vi "CANopen Emergency.vi"() -> ()   [LabVIEW 2016]
doc: "This example demonstrates how to read a CANopen emergency object."
uses:
  <vilib>/userdefined/High Color/nirio_resource_hc.ctl
  <vilib>/Platform/TimedLoop/XDataNode/timing_clust.ctl
  <vilib>/Platform/TimedLoop/XDataNode/nitl_modes.ctl
  <vilib>/Platform/TimedLoop/XDataNode/wakeup.ctl
  <vilib>/FPGAPlugInAG/cRIO-9033/niLvFpga_Open_cRIO-9033.vi
  <vilib>/rvi/interface/common/dynamic/niFpgaDynamicAddResources.vi
  <vilib>/CANopenLib/CANOPEN.llb/CANopen Interface Create.vi
  <vilib>/CANopenLib/CANOPEN.llb/CANopen Emergency Create.vi
  <vilib>/CANopenLib/CANOPEN.llb/CANopen Emergency Start.vi
  <vilib>/CANopenLib/CANOPEN.llb/CANopen Emergency Read.vi
  <vilib>/CANopenLib/CANOPEN.llb/CANopen Emergency Close.vi
  <vilib>/CANopenLib/CANOPEN.llb/CANopen Interface Close.vi
  <vilib>/FPGAPlugInAG/Dynamic/niLvFpga_Close_Dynamic.vi
  <vilib>/rvi/interface/nirviOpenFPGA/nirviOpenFPGA.xnode
  FPGA Bitfiles/project_FPGATarget_MainFPGA_S9ZLErdeBuw.lvbitx
  FPGA/MainFPGA.vi
  <vilib>/Platform/TimedLoop/XDataNode/XDataNode.xnode
  <vilib>/rvi/interface/nirviCloseFPGA/nirviCloseFPGA.xnode
  <vilib>/Platform/TimedLoop/XDataNode/XDNodeRunTimeDep.lvlib
panel:
  in  "error in":errorcluster
  out "emergency message":T1
  out "Is new?":bool
  out "timestamp":timestamp
  in  "stop":bool
  in  "period (ms)":i64=10
  in  "queue size":u16
  in  "node-ID":u8=1 min=1 max=127 step=1
  in  "baud rate":u32(ring)=2 items=["1 Mbit/s"=0, "800 kbit/s"=1, "500 kbit/s"=2, "250 kbit/s"=3, "125 kbit/s"=4, "50 kbit/s"=6, "20 kbit/s"=7, "10 kbit/s"=8]
  in  "CANopen interface":u32(ring) items=["CANopen01", "CANopen02", "CANopen03", "CANopen04", "CANopen05", "CANopen06", "CANopen07", "CANopen08", "CANopen09", "CANopen10", "CANopen11", "CANopen12", "CANopen13", "CANopen14", "CANopen15", "CANopen16", "CANopen17", "CANopen18", "CANopen19", "CANopen20", "CANopen21", "CANopen22", "CANopen23", "CANopen24", "CANopen25", "CANopen26", "CANopen27", "CANopen28", "CANopen29", "CANopen30", "CANopen31", "CANopen32"]
  # "Overview: This example demonstrates how to read a CANopen Emergency object.\nRequirements: Connect CANopen module with a slave device. \nInstructions: \n1. Specify the values of CANopen interface, baud rate of the CANopen interface, node-ID of the slave device and\n    queue size of Emergency object. \n2. Run this VI.\n3. Click STOP to stop the VI."
  # "Create CANopen interface and Emergency object"
  # "Read Emergency messages"
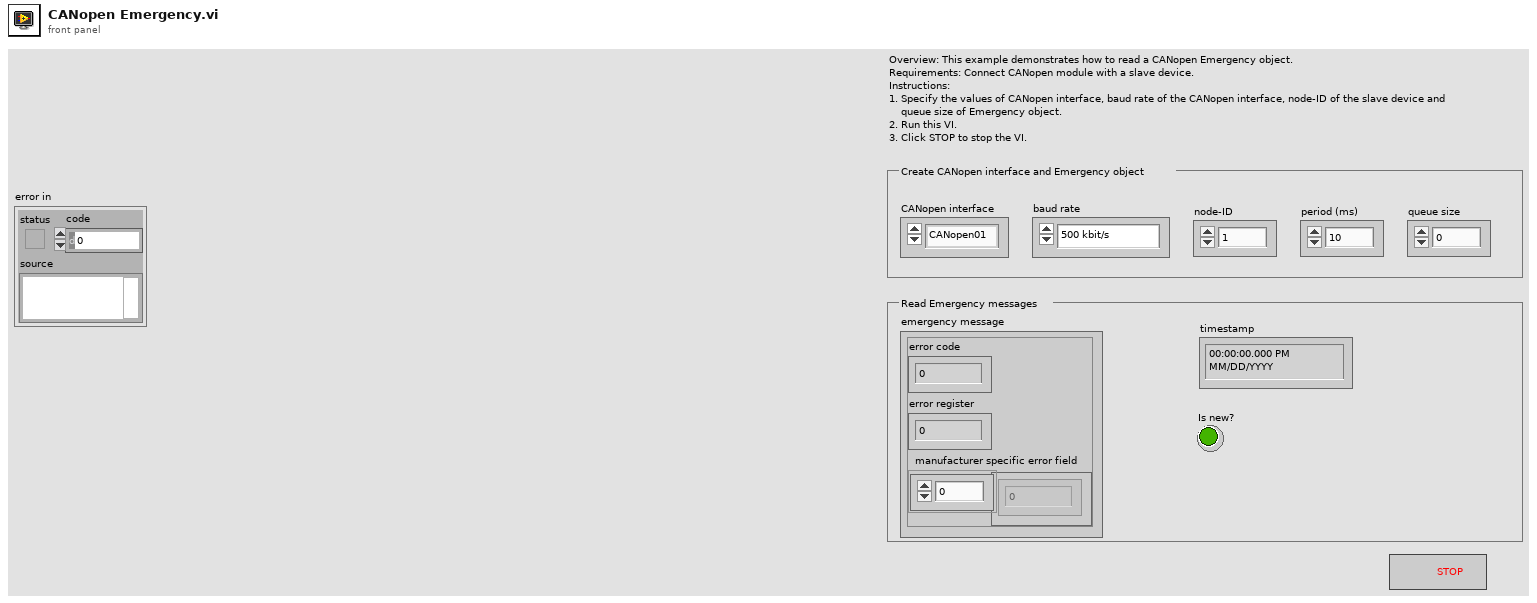
[diagram p1: front panel]
types:
  T1 = cluster{"error code":dbl, "error register":dbl, "manufacturer specific error field":dbl[]}
  T2 = typedef "nirio_resource_hc.ctl" = tag
  T3 = typedef "XDNodeRunTimeDep.lvlib/timing_clust.ctl" = cluster{"Expected End [f-1]":u64, "Actual End [f-1]":u64, "Finished Late? [f-1]":bool, "Expected End [i-1]":u64, "Actual End [i-1]":u64, "Finished Late? [i-1]":bool, "Expected Start [i]":u64, "Actual Start [i]":u64, "Expected Start [f]":u64, "Actual Start [f]":u64, "Source Name":string, "Structure Name":string, "Period":i64, "Deadline":i64, "Offset":i64, "Start":i64, "Priority":i32, "Timeout":i32, "Mode":T4, "Wakeup Reason":T5, "Error":errorcluster, "Source Type":string, "Secondary Source Type":string, "Global End Time":u64, "Global Start Time":u64, "Frame Duration":u64, "Iteration Duration":u64, "Assigned CPU":i32, "I/O Scan Engine Mode":u32}
  T4 = typedef "XDNodeRunTimeDep.lvlib/nitl_modes.ctl" = enum32{"No Change", "Process missed periods, maintain original phase", "Discard missed periods, maintain original phase", "Process missed periods, ignore original phase", "Discard missed periods, ignore original phase"}
  T5 = typedef "XDNodeRunTimeDep.lvlib/wakeup.ctl" = enum32{"Normal", "Aborted", "Asynchronous wakeup", "Timing source error", "Timed loop error", "Timeout"}
  T6 = cluster{"error code":u16, "error register":u8, "manufacturer specific error field":u8[]}
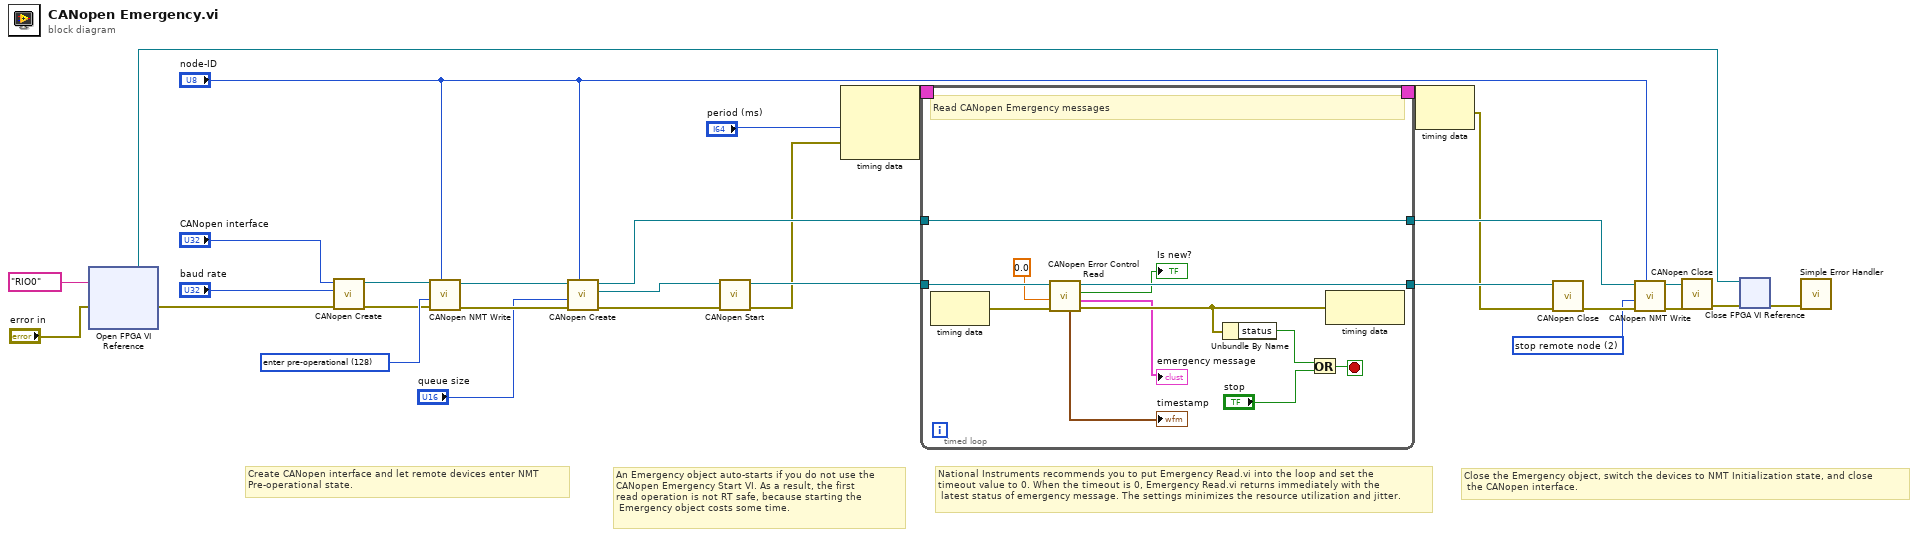
[diagram p0: block diagram]
diagram:
  w13 = u16 2 items=["start remote node"=1, "stop remote node"=2, "enter pre-operational"=128, "reset node"=129, "reset communication"=130] ("command")
  w24 = u16 128 items=["start remote node"=1, "stop remote node"=2, "enter pre-operational"=128, "reset node"=129, "reset communication"=130] ("command")
  # "An Emergency object auto-starts if you do not use the \nCANopen Emergency Start VI. As a result, the first \nread operation is not RT safe, because starting the\n Emergency object costs some time."
  # "Close the Emergency object, switch the devices to NMT Initialization state, and close\n the CANopen interface."
  # "Create CANopen interface and let remote devices enter NMT\nPre-operational state."
  # "National Instruments recommends you to put Emergency Read.vi into the loop and set the \ntimeout value to 0. When the timeout is 0, Emergency Read.vi returns immediately with the\n latest status of emergency message. The settings minimizes the resource utilization and jitter."
  n1 = xnode ("Open FPGA VI Reference")("error in"="error in", "resource name"=T2 "RIO0") -> ("FPGA VI Reference Out"=w1:refnum<k20>, "error out"=w4:errorcluster)
  n2 = call-poly <vilib>:"CANopen Create.vi"("error in (no error)"=w4, "baud rate"="baud rate", "interface name"="CANopen interface") -> ("error out"=w23:errorcluster, "interface object out"=w22:refnum<k20>)  [unwired: 7 in]
  n3 = call <vilib>:"CANopen NMT Write.vi"("node-ID (0)"="node-ID", "error in (no error)"=w23, "command"=w24, "interface object in"=w22) -> ("error out"=w27:errorcluster, "interface object out"=w28:refnum<k20>)  [unwired: 6 in]
  n4 = call-poly <vilib>:"CANopen Create.vi"("node-ID"="node-ID", "error in (no error)"=w27, "buffer size (0)"="queue size", "interface object in"=w28) -> ("error out"=w12:errorcluster, "emergency object out"=w11:refnum<k20>, "interface object out"=w15:refnum<k20>)  [unwired: 5 in]
  n5 = call-poly <vilib>:"CANopen Start.vi"("error in (no error)"=w12, "emergency object in"=w11) -> ("error out"=w9:errorcluster, "emergency object out"=w19:refnum<k20>)  [unwired: 8 in]
  n6 = node-c288("period (ms)", w9) -> (w30:T3)  [unwired: 1 in]
  n7 = timed-loop {
    tunnel: w19 -> [w41]
    tunnel: [w40] -> w20
    tunnel: w15 -> [w34]
    tunnel: [w34] -> w14
    timing: w30 -> [_]
    timing-out: [_] -> w29
    stop <- w37 stop-if-true
    # "Read CANopen Emergency messages"
    n8 = node-c288() -> (w33:errorcluster)  [unwired: 1 in]
    n9 = call-poly <vilib>:"CANopen Error Control Read.vi"("error in (no error)"=w33, "timeout (0s)"=0.0 ("timeout(0)"), "emergency object in"=w41) -> ("error out"=w32:errorcluster, "emergency message"=→"emergency message":T6, "new message?"=→"Is new?":bool, "emergency object out"=w40:refnum<k20>, "timestamp"=→"timestamp":timestamp)  [unwired: 4 in]
    n10 = Unbundle By Name(w32) -> ("status"=w35:bool)
    n11 = Or(x=w35, y="stop") -> (x .or. y?=w37:bool)
    n12 = node-c288(w32) -> ()  [unwired: 1 out]
  }
  n13 = node-c288(w29) -> (w8:errorcluster)
  n14 = call-poly <vilib>:"CANopen Close.vi"("error in (no error)"=w8, "emergency object in"=w20) -> ("error out"=w16:errorcluster)  [unwired: 9 in]
  n15 = call <vilib>:"CANopen NMT Write.vi"("node-ID (0)"="node-ID", "error in (no error)"=w16, "command"=w13, "interface object in"=w14) -> ("error out"=w18:errorcluster, "interface object out"=w17:refnum<k20>)  [unwired: 6 in]
  n16 = call-poly <vilib>:"CANopen Close.vi"("error in (no error)"=w18, "interface object in"=w17) -> ("error out"=w3:errorcluster)  [unwired: 9 in]
  n17 = xnode "Close FPGA VI Reference"("FPGA VI Reference In"=w1, "error in"=w3) -> ("error out"=w2:errorcluster)
  n18 = call <vilib>:"Simple Error Handler.vi"("error in (no error)"=w2) -> ()  [unwired: 4 in, 5 out]
